vi "LaserCal-Save Data (I-O).vi"(0 "System ID":T1, 7 "I-O Data":T2, 11 "error in (no error)":errorcluster) -> (15 "error out":errorcluster)   [LabVIEW 2015]
uses:
  Typedefs/LaserCal-Data (I-O).ctl
  Typedefs/LaserCal-System ID.ctl
panel:
  in  "Laser Calibration File":T3
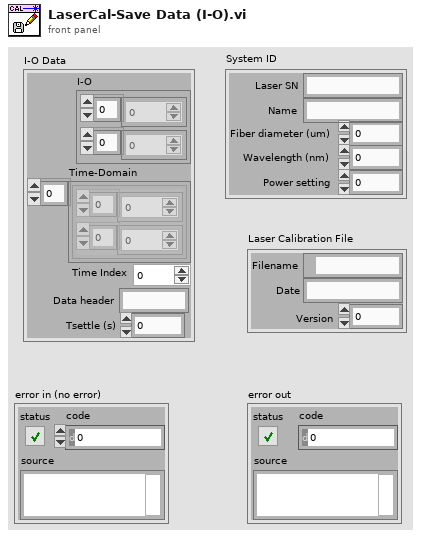
[diagram p1: front panel]
types:
  T1 = typedef "LaserCal-System ID.ctl" = cluster{"Name":string, "Laser SN":string, "Wavelength (nm)":dbl, "Fiber diameter (um)":dbl, "Power setting":dbl}
  T2 = typedef "LaserCal-Data (I-O).ctl" = cluster{"I-O":cluster{dbl[], dbl[]}, "Time-Domain":cluster{dbl[], dbl[]}[], "Time Index":i32, "Data header":string, "Tsettle (s)":dbl}
  T3 = cluster{"Filename":path, "Date":string, "Version":i32}
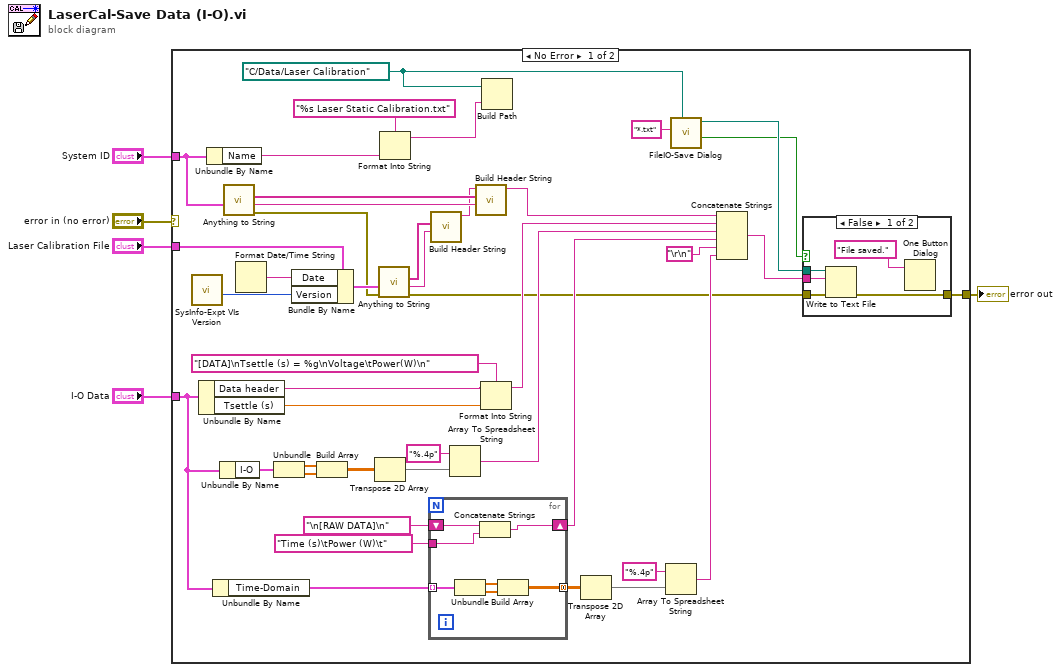
[diagram p0: block diagram]
diagram:
  n1 = case shown="No Error" "error in (no error)" {
    selector: "error in (no error)" -> [_ w62]
    tunnel: [w23 w62] -> w5
    tunnel: "Laser Calibration File" -> [w46 _]
    tunnel: "I-O Data" -> [w21 _]
    tunnel: "System ID" -> [w27 _]
    frame No Error {
      w10 = path "C:/Data/Laser Calibration"
      n2 = call "SysInfo-Expt VIs Version.vi"() -> ("Expt VIs Version out"=w47:i32)  [unwired: 11 in]
      n3 = Unbundle By Name(w21) -> ("Data header"=w35:string, "Tsettle (s)"=w36:dbl)
      n4 = Unbundle By Name(w27) -> ("Name"=w26:string)
      n5 = Unbundle By Name(w21) -> ("Time-Domain"=w20:cluster{dbl[], dbl[]}[])
      n6 = Unbundle By Name(w21) -> ("I-O"=w42:cluster{dbl[], dbl[]})
      n7 = call "Anything to String.vi"("Anything"=w27) -> ("Error Out"=w31:errorcluster, "Section"=w32:string, "Strings[]"=w30:string[])  [unwired: 8 in]
      n8 = Format Date/Time String() -> (date/time string=w48:string)  [unwired: 3 in]
      n9 = Unbundle(w42) -> (w41:dbl[], w40:dbl[])
      n10 = Bundle By Name(cluster=w46, "Date"=w48, "Version"=w47) -> (w45:T3)
      n11 = Build Array(w41, w40) -> (w39:dbl[][])
      n12 = Transpose 2D Array(2D array=w39) -> (transposed array=w12:dbl[][])
      n13 = call "Anything to String.vi"("Error In"=w31, "Anything"=w45) -> ("Error Out"=w8:errorcluster, "Section"=w43:string, "Strings[]"=w44:string[])  [unwired: 7 in]
      n14 = Format Into String(format string="%s Laser Static Calibration.txt", w26) -> (resulting string=w24:string)  [unwired: 2 in, 1 out]
      n15 = for {
        tunnel: w20 -> [w58] mode=indexing
        shift-right: [w59] -> w15
        shift-left: "\n[RAW DATA]\n" -> [w61]
        tunnel: "Time (s)\tPower (W)\t" -> [w60]
        tunnel: [w55] -> w16 mode=concatenating
        n16 = Unbundle(w58) -> (w57:dbl[], w56:dbl[])
        n17 = Concatenate Strings(w61, w60) -> (w59:string)
        n18 = Build Array(w57, w56) -> (w55:dbl[][])
      }
      n19 = call "Build Header String.vi"("Section"=w43, "Strings[]"=w44) -> ("Header out"=w29:string)  [unwired: 9 in]
      n20 = Array To Spreadsheet String(array=w12, 3:"%.4p" ("format string")) -> (spreadsheet string=w33:string)  [unwired: 1 in]
      n21 = call "Build Header String.vi"("Section"=w32, "Strings[]"=w30, "Header in"=w29) -> ("Header out"=w28:string)  [unwired: 8 in]
      n22 = Format Into String(format string="[DATA]\nTsettle (s) = %g\nVoltage\tPower(W)\n", initial string=w35, w36) -> (resulting string=w34:string)  [unwired: 1 in, 1 out]
      n23 = Build Path(base path=w10, name or relative path=w24) -> ()  [unwired: 1 out]
      n24 = Transpose 2D Array(2D array=w16) -> (transposed array=w11:dbl[][])
      n25 = Array To Spreadsheet String(array=w11, 3:"%.4p" ("format string")) -> (spreadsheet string=w13:string)  [unwired: 1 in]
      n26 = call "FileIO-Save Dialog.vi"("Default Folder"=w10, "pattern (all files)"="*.txt") -> ("cancelled"=w7:bool, "selected path"=w9:path)  [unwired: 7 in, 1 out]
      n27 = Concatenate Strings(w28, w34, w33, w15, "\r\n", w13) -> (w22:string)
      n28 = case shown="False" w7 {
        tunnel: [w53 w54] -> w23
        tunnel: w22 -> [w52 _]
        tunnel: w9 -> [w51 _]
        tunnel: w8 -> [w50 w54]
        frame False {
          n29 = Write to Text File(file (use dialog)=w51, text=w52, error in=w50) -> (error out=w53:errorcluster)  [unwired: 1 in, 2 out]
          n30 = One Button Dialog(message="File saved.") -> ()  [unwired: 1 in, 1 out]
        }
        frame True {
        }
      }
    }
    frame Error {
    }
  }
  "error out" <- w5
